vi "Fade-In VI.vi"(4 "Close on Fade-Out [T]":bool, 5 "Delay (ms) [0]":i32, 6 "Fade Direction [Fade In]":enum16{"Fade In", "Fade Out"}(ring), 7 "Fade-in time (ms) [500]":u32=500, 10 "stop notifier":refnum<notifier>, 11 "VI Ref":refnum<vi>) -> ()   [LabVIEW 2017]
doc: "Opens VI front panel and fades in over time indicated by fade-in time. This VI can be called dynamiucally to allow the fade-in to happen even while the calling VI is being moved around.\n\nThe delay is how long you want before the VI begins to open. This is helpful for tip strips. Delay is cancleable by notifier."
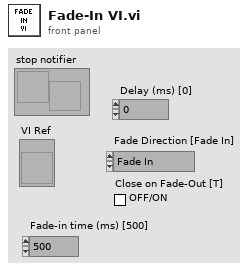
[diagram p1: front panel]
types:
  T1 = enum32{"Invalid", "Standard", "Closed", "Hidden", "Minimized", "Maximized"}
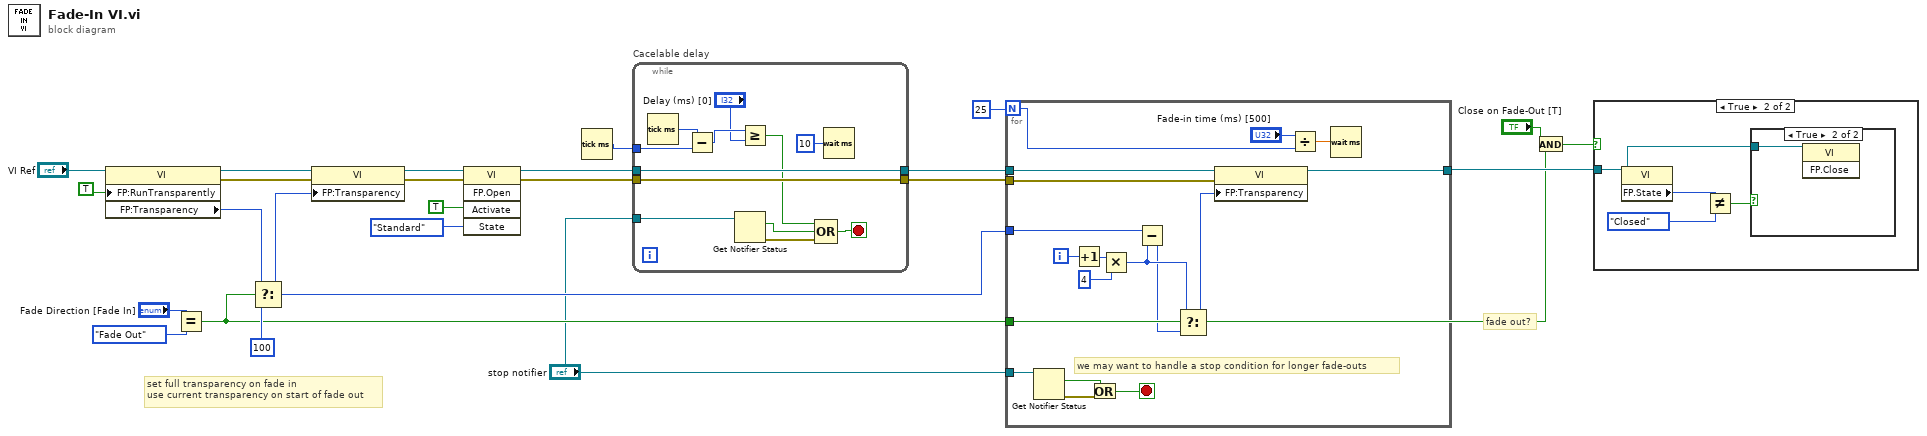
[diagram p0: block diagram]
diagram:
  # "fade out?"
  # "set full transparency on fade in\nuse current transparency on start of fade out"
  n1 = property class="VI"(reference="VI Ref", "FP:RunTransparently"=TRUE ("Front Panel Window:Run VI Transparently")) -> (reference out=w15:refnum<vi>, error out=w16:errorcluster, "FP:Transparency"=w12:u8)  [unwired: 1 in]
  n2 = Equal?(x="Fade Direction [Fade In]", y=enum16{"Fade In", "Fade Out"}."Fade Out" ("Fade Direction")) -> (x = y?=w9:bool)
  n3 = Select(t=w12, s=w9, f=u8 100 ("Front Panel Window:Transparency")) -> (s? t:f=w10:u8)
  n4 = property class="VI"(reference=w15, error in=w16, "FP:Transparency"=w10) -> (reference out=w13:refnum<vi>, error out=w14:errorcluster)
  n5 = invoke class="VI" method="FP.Open"(reference=w13, error in=w14, "Activate"=TRUE, "State"=T1."Standard") -> (reference out=w6:refnum<vi>, error out=w5:errorcluster)  [unwired: 1 in, 3 out]
  n6 = Tick Count (ms)() -> (millisecond timer value=w1:u32)
  n7 = while "Cacelable delay" {
    tunnel: [w36] -> w4
    tunnel: w6 -> [w36]
    tunnel: [w35] -> w3
    tunnel: w5 -> [w35]
    tunnel: "stop notifier" -> [w33]
    tunnel: w1 -> [w31]
    stop <- w27 stop-if-true
    n8 = Tick Count (ms)() -> (millisecond timer value=w32:u32)
    n9 = Subtract(x=w32, y=w31) -> (x-y=w26:u32)
    n10 = Get Notifier Status(notifier=w33) -> (current notification=w29:bool, error out=w30:errorcluster)  [unwired: 1 in, 3 out]
    n11 = Greater Or Equal?(x=w26, y="Delay (ms) [0]") -> (x >= y?=w28:bool)
    n12 = Compound Arithmetic op=OR(w28, w29, w30) -> (w27:bool)
    n13 = Wait (ms)(milliseconds to wait=u32 10) -> ()  [unwired: 1 out]
  }
  n14 = for {
    N: 25 -> [w48]
    tunnel: w4 -> [w54]
    tunnel: w3 -> [w47]
    tunnel: w9 -> [w46]
    tunnel: "stop notifier" -> [w42]
    tunnel: [w38] -> w18
    tunnel: w10 -> [w37]
    i -> [w53]
    stop <- w39 stop-if-true
    # "we may want to handle a stop condition for longer fade-outs"
    n15 = Get Notifier Status(notifier=w42) -> (current notification=w40:bool, error out=w41:errorcluster)  [unwired: 1 in, 3 out]
    n16 = Increment(x=w53) -> (x+1=w49:i32)
    n17 = Or(x=w40, y=w41) -> (x .or. y?=w39:bool)
    n18 = Multiply(x=w49, y=4) -> (x*y=w45:i32)
    n19 = Subtract(x=w37, y=w45) -> (x-y=w44:i32)
    n20 = Select(t=w45, s=w46, f=w44) -> (s? t:f=w43:i32)
    n21 = property class="VI"(reference=w54, error in=w47, "FP:Transparency"=w43) -> (reference out=w38:refnum<vi>)  [unwired: 1 out]
    n22 = Divide(x="Fade-in time (ms) [500]", y=w48) -> (x/y=w50:dbl)
    n23 = Wait (ms)(milliseconds to wait=w50) -> ()  [unwired: 1 out]
  }
  n24 = And(x="Close on Fade-Out [T]", y=w9) -> (x .and. y?=w7:bool)
  n25 = case shown="True" w7 {
    tunnel: w18 -> [_ w55]
    frame False {
    }
    frame True {
      n26 = property class="VI"(reference=w55) -> ("FP.State"=w58:T1)  [unwired: 1 in, 2 out]
      n27 = Not Equal?(x=w58, y=T1."Closed" ("Front Panel Window:State")) -> (x != y?=w56:bool)
      n28 = case shown="True" w56 {
        tunnel: w55 -> [_ w59]
        frame False {
        }
        frame True {
          n29 = invoke class="VI" method="FP.Close"(reference=w59) -> ()  [unwired: 2 in, 3 out]
        }
      }
    }
  }
